vi "SetMatlabTempParamData.vi"(8 "index in":dbl=-1.0, 10 "Matlab param data":T1[](array[typedef]), 11 "ExperimentID":string) -> (3 "index out":dbl)   [LabVIEW 2017]
uses:
  Types/MatlabDataBundle.ctl
  Types/MatlabDataType.ctl
  <vilib>/Utility/Data Type/Type Definitions/Data Type.ctl
  <vilib>/Utility/Data Type/NI_Data Type.lvlib
panel:
  out "String":string
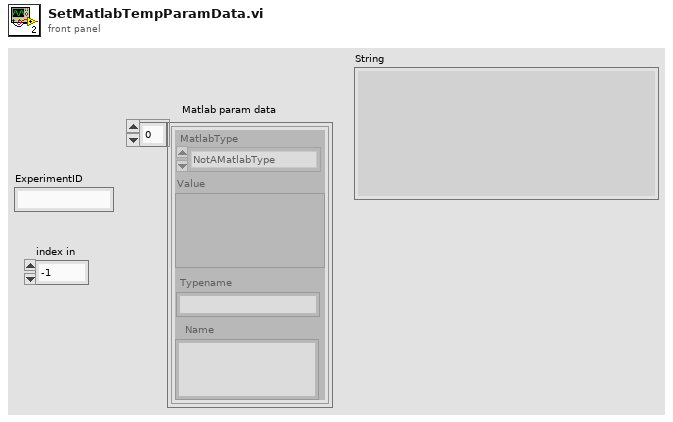
[diagram p1: front panel]
types:
  T1 = typedef "MatlabDataBundle.ctl" = cluster{"MatlabType":T2, "Value":variant, "Name":string, "Typename":string}
  T2 = typedef "MatlabDataType.ctl" = enum16{"NotAMatlabType", "Real", "Complex", "String", "Boolean"}
  T3 = typedef "NI_Data Type.lvlib/Data Type.ctl" = enum8{"Invalid Type", "Void", "I8", "I16", "I32", "I64", "U8", "U16", "U32", "U64", "Single Float", "Double Float", "Extended Float", "Single Complex", "Double Complex", "Extended Complex", "Enum U8", "Enum U16", "Enum U32", "Enum U64", "Single Float With Unit", "Double Float With Unit", "Extended Float With Unit", "Single Complex with Unit", "Double Complex with Unit", "Extended Complex with Unit", "Boolean", "String", "Path", "Picture", "Tag", "Array", "Cluster", "Variant", "LV Variant", "Waveform", "Timestamp", "Digital Waveform", "Digital Data", "ExpressData", "Refnum", "External Data", "VI", "Poly VI", "LabVIEW Class Instance", "Fixed Point"}
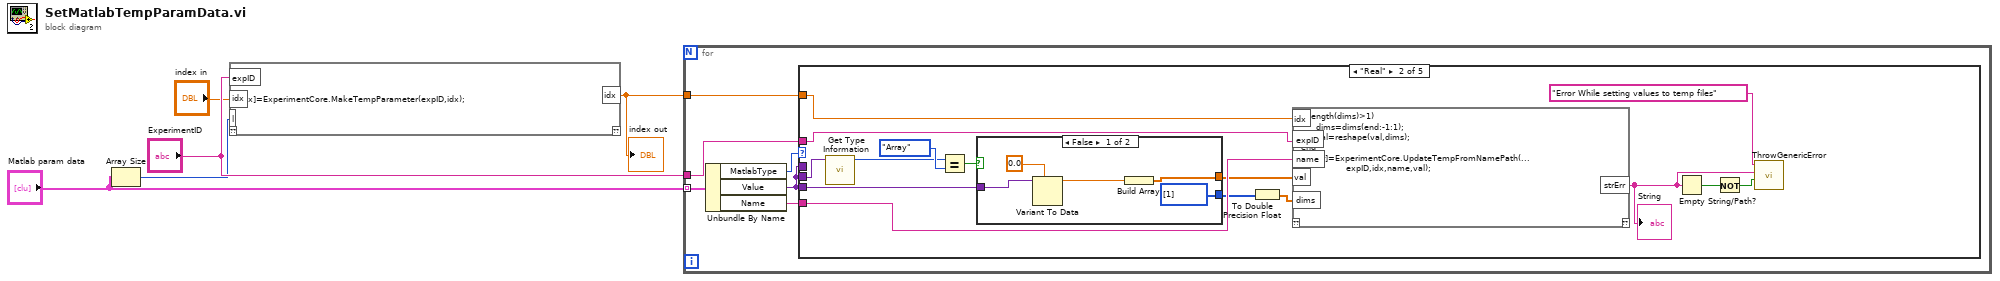
[diagram p0: block diagram]
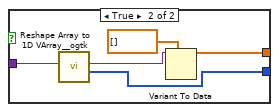
[diagram p3: hidden frame]
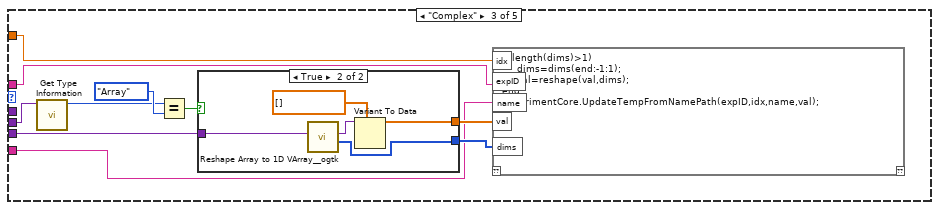
[diagram p4: hidden frame]
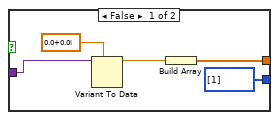
[diagram p5: hidden frame]
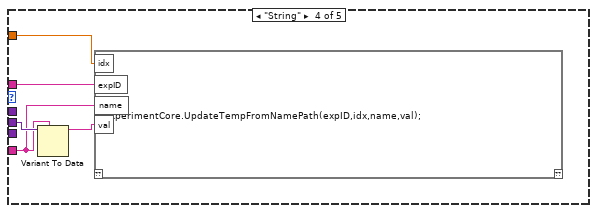
[diagram p6: hidden frame]
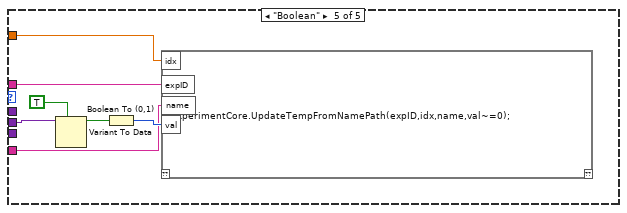
[diagram p7: hidden frame]
diagram:
  n1 = Array Size(array="Matlab param data") -> (size(s)=w1:i32)
  n2 = script code="[idx]=ExperimentCore.MakeTempParameter(expID,idx);"("expID"="ExperimentID", "idx"="index in", "l"=w1) -> ("idx"=w3:dbl)  [unwired: 1 in, 1 out]
  "index out" <- w3
  n3 = for {
    tunnel: "Matlab param data" -> [w10] mode=indexing
    tunnel: "ExperimentID" -> [w11]
    tunnel: w3 -> [w6]
    n4 = Unbundle By Name(w10) -> ("MatlabType"=w9:T2, "Value"=w7:variant, "Name"=w8:string)
    n5 = case shown="\"Real\"" w9 {
      tunnel: w11 -> [_ w26 w39 w60 w65]
      tunnel: w7 -> [_ w24 w46 w61 w64]
      tunnel: w8 -> [_ w25 w37 w59 w63]
      tunnel: w7 -> [_ _ _ _ _]
      tunnel: w7 -> [_ w19 w42 _ _]
      tunnel: w6 -> [_ w16 w38 w57 w62]
      frame "NotAMatlabType", Default {
      }
      frame "Real" {
        n6 = call <vilib>:"Get Type Information.vi"("Variant"=w24) -> ("Type"=w22:T3)  [unwired: 6 in, 4 out]
        n7 = Equal?(x=w22, y=Data_Type."Array" ("Type")) -> (x = y?=w21:bool)
        n8 = case shown="False" w21 {
          tunnel: [w29 w35] -> w20
          tunnel: w19 -> [w27 w34]
          tunnel: [u32[] [1] ("Size(s)") w33] -> w18
          frame False {
            n9 = Variant To Data(type=0.0, Variant=w27) -> (data=w30:dbl)  [unwired: 1 in, 1 out]
            n10 = Build Array(w30) -> (w29:dbl[])
          }
          frame True {
            n11 = call <userlib>:"Reshape Array to 1D VArray__ogtk.vi"("MultiD Array"=w34) -> ("Size(s)"=w33:u32[], "1D VArray"=w32:variant)  [unwired: 8 in, 1 out]
            n12 = Variant To Data(type=dbl[] [], Variant=w32) -> (data=w35:dbl[])  [unwired: 1 in, 1 out]
          }
        }
        n13 = To Double Precision Float(number=w18) -> (double precision float=w17:dbl[])
        n14 = script code="if(length(dims)>1)\n     dims=dims(end:-1:1);\n     val=reshape(val,dims);\nend\n[strErr]=ExperimentCore.UpdateTempFromNamePath(...\n               expID,idx,name,val);"("expID"=w26, "name"=w25, "val"=w20, "dims"=w17, "idx"=w16) -> ("strErr"=w13:string)  [unwired: 1 in, 1 out]
        "String" <- w13
        n15 = Empty String/Path?(string/path=w13) -> (empty?=w15:bool)
        n16 = Not(x=w15) -> (.not. x?=w12:bool)
        n17 = call "ThrowGenericError.vi"("Invoke?"=w12, "Error info"=w13, "TheError"="Error While setting values to temp files") -> ()  [unwired: 8 in, 1 out]
      }
      frame "Complex" {
        n18 = call <vilib>:"Get Type Information.vi"("Variant"=w46) -> ("Type"=w44:T3)  [unwired: 6 in, 4 out]
        n19 = Equal?(x=w44, y=Data_Type."Array" ("Type")) -> (x = y?=w43:bool)
        n20 = case shown="True" w43 {
          tunnel: [w50 w55] -> w40
          tunnel: w42 -> [w48 w54]
          tunnel: [u32[] [1] ("Size(s)") w53] -> w41
          frame False {
            n21 = Variant To Data(type=cdb 0.0+0.0i, Variant=w48) -> (data=w51:cdb)  [unwired: 1 in, 1 out]
            n22 = Build Array(w51) -> (w50:cdb[])
          }
          frame True {
            n23 = call <userlib>:"Reshape Array to 1D VArray__ogtk.vi"("MultiD Array"=w54) -> ("Size(s)"=w53:u32[], "1D VArray"=w52:variant)  [unwired: 8 in, 1 out]
            n24 = Variant To Data(type=cdb[] [], Variant=w52) -> (data=w55:cdb[])  [unwired: 1 in, 1 out]
          }
        }
        n25 = script code="if(length(dims)>1)\n     dims=dims(end:-1:1);\n     val=reshape(val,dims);\nend\nExperimentCore.UpdateTempFromNamePath(expID,idx,name,val);"("expID"=w39, "name"=w37, "val"=w40, "dims"=w41, "idx"=w38) -> ()  [unwired: 1 in, 1 out]
      }
      frame "String" {
        n26 = Variant To Data(type=w59, Variant=w61) -> (data=w58:string)  [unwired: 1 in, 1 out]
        n27 = script code="ExperimentCore.UpdateTempFromNamePath(expID,idx,name,val);"("expID"=w60, "name"=w59, "val"=w58, "idx"=w57) -> ()  [unwired: 1 in, 1 out]
      }
      frame "Boolean" {
        n28 = Variant To Data(type=TRUE, Variant=w64) -> (data=w67:bool)  [unwired: 1 in, 1 out]
        n29 = Boolean To (0,1)(Boolean=w67) -> (0, 1=w66:i16)
        n30 = script code="ExperimentCore.UpdateTempFromNamePath(expID,idx,name,val~=0);"("expID"=w65, "name"=w63, "val"=w66, "idx"=w62) -> ()  [unwired: 1 in, 1 out]
      }
    }
  }
